vi "Test Launch Runner with Test Case.vi"(8 "error in (no error)":errorcluster, 11 "Test Runner Test in":refnum<class "Test Runner Test.lvclass">) -> (0 "error out":errorcluster, 3 "Test Runner Test out":refnum<class "Test Runner Test.lvclass">)   [LabVIEW 2020, in "Test Runner Test.lvclass"]
uses:
  Test Runner Test.lvclass
  C:/Git/astemes-lunit/source/Core/Result Observer/Result Observer.lvclass
  Framework/Single Thread Test Runner/Single Thread Test Runner.lvclass
  Core/LUnit Test Suite/LUnit Test Suite.lvclass
  C:/Git/astemes-lunit/source/Core/Runnable/Runnable.lvclass
  Test Runner Test.lvclass/Test Runner Test.ctl
  C:/Program Files (x86)/National Instruments/LabVIEW 2020/vi.lib/Astemes/LUnit/Test Case.lvclass
  C:/Git/astemes-lunit/source/Tests/Test Runner Test/Test Runner Test.lvclass
  C:/Git/astemes-lunit/source/Core/LUnit Test Suite/LUnit Test Suite.lvclass
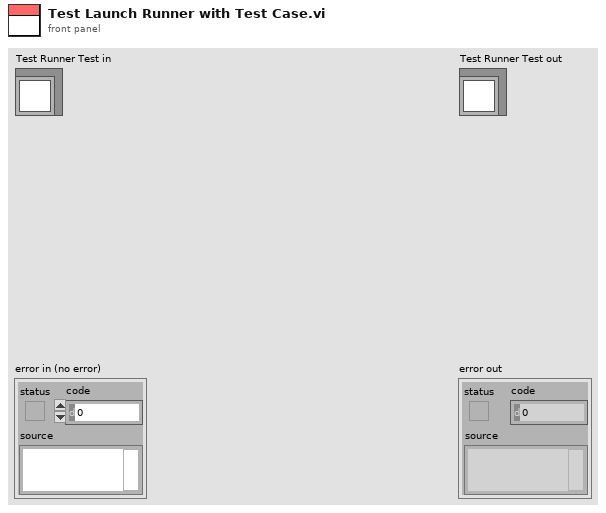
[diagram p1: front panel]
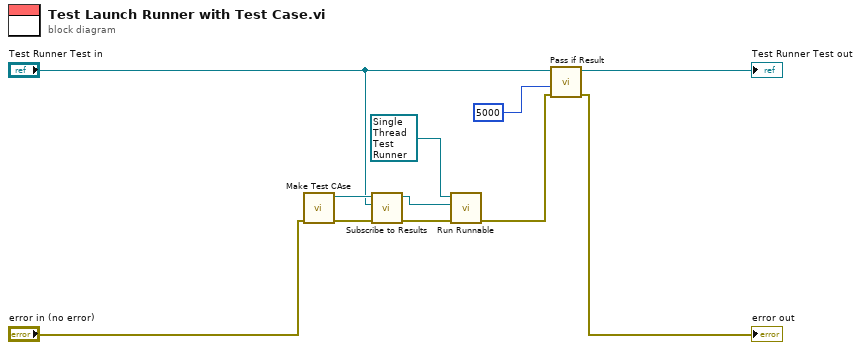
[diagram p0: block diagram]
diagram:
  n1 = call "Make Test CAse.vi"("error in (no error)"="error in (no error)") -> ("error out"=w10:errorcluster, "LUnit Test Suite V2 out"=w11:refnum<class "LUnit Test Suite.lvclass">)  [unwired: 9 in]
  n2 = call-dynamic "Subscribe to Results.vi"("error in (no error)"=w10, "Result Observer"="Test Runner Test in", "LUnit Test Suite In"=w11) -> ("error out"=w6:errorcluster, "LUnit Test Suite Out"=w7:refnum<class "LUnit Test Suite.lvclass">)  [unwired: 7 in]
  n3 = call-dynamic "Run Runnable.vi"("error in (no error)"=w6, "Runnable"=w7, "Test Runner"=refnum<class "Single Thread Test Runner.lvclass"> refnum) -> ("error out"=w5:errorcluster)  [unwired: 8 in]
  n4 = call "Pass if Result.vi"("error in (no error)"=w5, "timeout in ms (0)"=5000, "Test Runner Test in"="Test Runner Test in") -> ("error out"=→"error out":errorcluster, "Test Runner Test out"=→"Test Runner Test out":refnum<class "Test Runner Test.lvclass">)  [unwired: 7 in]
